vi "Write Setpoint.vi"(7 "listen period":sgl=0.1, 8 "error in":errorcluster, 9 "Flow Unit":u8(ring)=57 items=["litres/minute"=17, "dubic meters/hour"=19, "litres/second"=24, "cubic meters/second"=28, "percent of flow range"=57, "grams/second"=70, "grams/minute"=71, "grams/hour"=72, "kilograms/second"=73, "kilograms/minute"=74, "kilograms/hour"=75, "pounds/second"=80, "pounds/minute"=81, "pounds/hour"=82, "cubic meters/minute"=131, "liters/hour"=138, "millimeters/second"=170, "milimeters/minute"=171, "millimeters/hour"=172, ""=0], 10 "Setpoint":sgl=80.0, 11 "Brooks MFC in":refnum<class "Brooks MFC.lvclass">) -> (0 "error out":errorcluster, 3 "Brooks MFC out":refnum<class "Brooks MFC.lvclass">)   [LabVIEW 2016, in "Brooks MFC.lvclass"]
uses:
  Brooks MFC.lvclass
  Brooks MFC.lvclass/Brooks MFC.ctl
  Instance           3 22Saved   Write Setpoint .vi
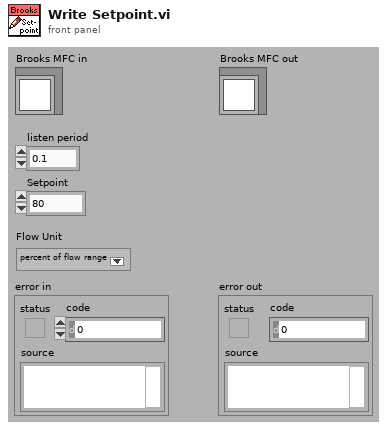
[diagram p1: front panel]
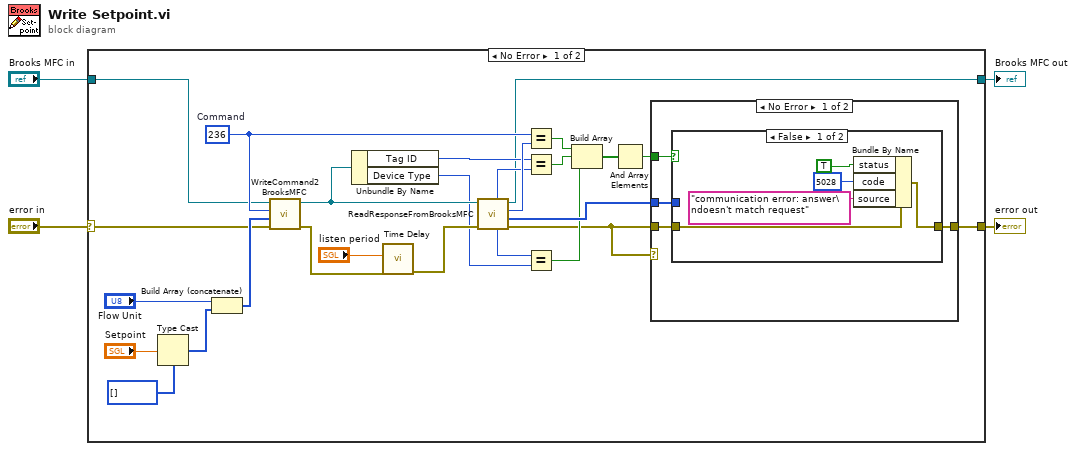
[diagram p0: block diagram]
diagram:
  n1 = case shown="No Error" "error in" {
    selector: "error in" -> [w7 w42]
    tunnel: "Brooks MFC in" -> [w8 w43]
    tunnel: [w6 w43] -> w2
    tunnel: [w5 w42] -> w1
    frame No Error {
      w14 = u8 236  # Command
      n2 = Type Cast(type=u8[] [] ("Unsigned 8 bit array"), x="Setpoint") -> (*(type *) &x=w15:u8[])
      n3 = Build Array (concatenate)("Flow Unit", w15) -> (w13:u8[])
      n4 = call "WriteCommand2BrooksMFC.vi"("error in"=w7, "Data"=w13, "Command"=w14, "Brooks MFC in"=w8) -> ("error out"=w28:errorcluster, "Brooks MFC out"=w11:refnum<class "Brooks MFC.lvclass">)  [unwired: 5 in, 1 out]
      n5 = Unbundle By Name(w11) -> ("Tag ID"=w10:u32, "Device Type"=w9:u8)
      n6 = call "Time Delay"("error in (no error)"=w28, "Delay Time (s)"="listen period") -> ("error out"=w26:errorcluster)  [unwired: 9 in]
      n7 = call "ReadResponseFromBrooksMFC.vi"("error in"=w26, "Brooks MFC in"=w11) -> ("error out"=w12:errorcluster, "Data"=w30:u8[], "Command"=w29:u8, "Brooks MFC out"=w6:refnum<class "Brooks MFC.lvclass">, "device type"=w24:u8, "tag ID"=w25:u32)  [unwired: 4 in]
      n8 = Equal?(x=w14, y=w29) -> (x = y?=w23:bool)
      n9 = Equal?(x=w10, y=w25) -> (x = y?=w22:bool)
      n10 = Equal?(x=w24, y=w9) -> (x = y?=w21:bool)
      n11 = Build Array(w23, w22, w21) -> (w20:bool[])
      n12 = And Array Elements(Boolean array=w20) -> (logical AND=w19:bool)
      n13 = case shown="No Error" w12 {
        tunnel: w12 -> [w34 w41]
        tunnel: w30 -> [w33 _]
        tunnel: [w32 w41] -> w5
        tunnel: w19 -> [w31 _]
        frame No Error {
          n14 = case shown="False" w31 {
            tunnel: w33 -> [_ _]
            tunnel: w34 -> [w36 w40]
            tunnel: [w35 w40] -> w32
            frame False {
              n15 = Bundle By Name(cluster=w36, "status"=TRUE ("Bundle Element"), "code"=5028 ("Bundle Element"), "source"="communication error: answer\ndoesn't match request" ("Bundle Element")) -> (w35:errorcluster)
            }
            frame True {
            }
          }
        }
        frame Error {
        }
      }
    }
    frame Error {
    }
  }
  "Brooks MFC out" <- w2
  "error out" <- w1
